vi "Get Lines Parameters.vi"(6 "P2 Y (unreleased)":refnum<class "1D Array f32.lvclass">, 8 "error in (no error)":errorcluster, 9 "P1 Y (unreleased)":refnum<class "1D Array f32.lvclass">, 10 "P2 X (unreleased)":refnum<class "1D Array f32.lvclass">, 11 "P1 X (unreleased)":refnum<class "1D Array f32.lvclass">) -> (0 "error out":errorcluster, 1 "Quadrant Correction X":refnum<class "1D Array f32.lvclass">, 2 "Direction Coefficients":refnum<class "1D Array f32.lvclass">, 3 "Quadrant Correction Y":refnum<class "1D Array f32.lvclass">, 5 "Length of Lines":refnum<class "1D Array f32.lvclass">, 7 "Is Row Major Line":refnum<class "1D Array binary.lvclass">)   [LabVIEW 2024, in "G2CPU Line Profile.lvlib"]
uses:
  G2CPU Line Profile.lvlib
  <vilib>/Natan Biesmans/G2CPU GPU and CPU HPC Toolkit/G2CPU Libraries/Arrays/1DArray/f32/1D Array f32.lvclass
  C:/Program Files/National Instruments/LabVIEW 2025/vi.lib/Natan Biesmans/G2CPU GPU and CPU HPC Toolkit/G2CPU Libraries/Arrays/Array/Array Prototype.lvclass
  <vilib>/Natan Biesmans/G2CPU GPU and CPU HPC Toolkit/G2CPU Libraries/Arrays/1DArray/binary/1D Array binary.lvclass
  cbe0f89a-fc6c-489f-bd70-ceba54479500.vi
  1a5ec087-74ba-4451-afc4-8685a5b5da5b.vi
  39281530-9ad4-4b96-9f34-9893a8ab4de5.vi
  7e7af70b-50f8-473b-bd23-2dd50eabd212.vi
  0e1627f4-ff60-46ab-8acd-18b1de2a0878.vi
  0517fff0-634e-4db0-931a-045051f9f055.vi
  a74614b9-8be0-4acb-b2b7-f56f2ea25a1a.vi
  cbe0f89a-fc6c-489f-bd70-ceba54479500.vi/1bf6e03b-eb75-45f6-9764-49dc38a3a024.vi
  cbe0f89a-fc6c-489f-bd70-ceba54479500.vi/2da4419f-02df-47a7-be00-1b7e0871fa33.vi
  1a5ec087-74ba-4451-afc4-8685a5b5da5b.vi/1bf6e03b-eb75-45f6-9764-49dc38a3a024.vi
  1a5ec087-74ba-4451-afc4-8685a5b5da5b.vi/2da4419f-02df-47a7-be00-1b7e0871fa33.vi
  39281530-9ad4-4b96-9f34-9893a8ab4de5.vi/def40612-844c-421c-bb75-87c330777b0b.vi
  7e7af70b-50f8-473b-bd23-2dd50eabd212.vi/def40612-844c-421c-bb75-87c330777b0b.vi
  0e1627f4-ff60-46ab-8acd-18b1de2a0878.vi/46771f49-eb1d-473b-8e81-f516cef50a4e.vi
  0e1627f4-ff60-46ab-8acd-18b1de2a0878.vi/dc76f8e4-64fa-456a-8549-7a4b6936c4c9.vi
  0e1627f4-ff60-46ab-8acd-18b1de2a0878.vi/7e60ddfb-e748-4c0c-85da-e395a1b7978d.vi
  0e1627f4-ff60-46ab-8acd-18b1de2a0878.vi/d2eceff7-f641-4ce4-acfa-e9e293a3c877.vi
  0e1627f4-ff60-46ab-8acd-18b1de2a0878.vi/b737122b-4036-448b-abd3-e2701355e828.vi
  0517fff0-634e-4db0-931a-045051f9f055.vi/494f1156-cf2e-4254-b6af-02aaeb6c0aff.vi
  0517fff0-634e-4db0-931a-045051f9f055.vi/44c17688-3442-4a50-bd81-3405ead58fa2.vi
  a74614b9-8be0-4acb-b2b7-f56f2ea25a1a.vi/b114fc2c-bc52-4e9d-afcd-b3046867ff8e.vi
  a74614b9-8be0-4acb-b2b7-f56f2ea25a1a.vi/ad131c31-fa70-445f-95fa-04e91a18ad4e.vi
  cbe0f89a-fc6c-489f-bd70-ceba54479500.vi/1bf6e03b-eb75-45f6-9764-49dc38a3a024.vi/3e802c67-fb96-46a3-ae13-4994a8508b4f.vi
  cbe0f89a-fc6c-489f-bd70-ceba54479500.vi/1bf6e03b-eb75-45f6-9764-49dc38a3a024.vi/5a50fc67-79e7-4972-80c2-92243cd53dd4.vi
  cbe0f89a-fc6c-489f-bd70-ceba54479500.vi/2da4419f-02df-47a7-be00-1b7e0871fa33.vi/730f6c57-5c0b-4ee9-b61e-75067b25222b.vi
  cbe0f89a-fc6c-489f-bd70-ceba54479500.vi/2da4419f-02df-47a7-be00-1b7e0871fa33.vi/096b8799-7810-404e-baca-ba9279cec4bd.vi
  cbe0f89a-fc6c-489f-bd70-ceba54479500.vi/2da4419f-02df-47a7-be00-1b7e0871fa33.vi/0f1a5a47-bcc5-4796-ac31-8dfcfbc0d7d1.vi
  cbe0f89a-fc6c-489f-bd70-ceba54479500.vi/2da4419f-02df-47a7-be00-1b7e0871fa33.vi/89f12e17-3330-4b72-ad8f-8dd636660732.vi
  1a5ec087-74ba-4451-afc4-8685a5b5da5b.vi/1bf6e03b-eb75-45f6-9764-49dc38a3a024.vi/3e802c67-fb96-46a3-ae13-4994a8508b4f.vi
  1a5ec087-74ba-4451-afc4-8685a5b5da5b.vi/1bf6e03b-eb75-45f6-9764-49dc38a3a024.vi/5a50fc67-79e7-4972-80c2-92243cd53dd4.vi
  1a5ec087-74ba-4451-afc4-8685a5b5da5b.vi/2da4419f-02df-47a7-be00-1b7e0871fa33.vi/730f6c57-5c0b-4ee9-b61e-75067b25222b.vi
  1a5ec087-74ba-4451-afc4-8685a5b5da5b.vi/2da4419f-02df-47a7-be00-1b7e0871fa33.vi/096b8799-7810-404e-baca-ba9279cec4bd.vi
  1a5ec087-74ba-4451-afc4-8685a5b5da5b.vi/2da4419f-02df-47a7-be00-1b7e0871fa33.vi/0f1a5a47-bcc5-4796-ac31-8dfcfbc0d7d1.vi
  1a5ec087-74ba-4451-afc4-8685a5b5da5b.vi/2da4419f-02df-47a7-be00-1b7e0871fa33.vi/89f12e17-3330-4b72-ad8f-8dd636660732.vi
  0e1627f4-ff60-46ab-8acd-18b1de2a0878.vi/dc76f8e4-64fa-456a-8549-7a4b6936c4c9.vi/3e802c67-fb96-46a3-ae13-4994a8508b4f.vi
  0e1627f4-ff60-46ab-8acd-18b1de2a0878.vi/dc76f8e4-64fa-456a-8549-7a4b6936c4c9.vi/5a50fc67-79e7-4972-80c2-92243cd53dd4.vi
  0517fff0-634e-4db0-931a-045051f9f055.vi/494f1156-cf2e-4254-b6af-02aaeb6c0aff.vi/edd31282-7992-4bba-af75-482693dee5e1.vi
  a74614b9-8be0-4acb-b2b7-f56f2ea25a1a.vi/b114fc2c-bc52-4e9d-afcd-b3046867ff8e.vi/edd31282-7992-4bba-af75-482693dee5e1.vi
  a74614b9-8be0-4acb-b2b7-f56f2ea25a1a.vi/ad131c31-fa70-445f-95fa-04e91a18ad4e.vi/730f6c57-5c0b-4ee9-b61e-75067b25222b.vi
  a74614b9-8be0-4acb-b2b7-f56f2ea25a1a.vi/ad131c31-fa70-445f-95fa-04e91a18ad4e.vi/096b8799-7810-404e-baca-ba9279cec4bd.vi
  a74614b9-8be0-4acb-b2b7-f56f2ea25a1a.vi/ad131c31-fa70-445f-95fa-04e91a18ad4e.vi/0f1a5a47-bcc5-4796-ac31-8dfcfbc0d7d1.vi
  a74614b9-8be0-4acb-b2b7-f56f2ea25a1a.vi/ad131c31-fa70-445f-95fa-04e91a18ad4e.vi/89f12e17-3330-4b72-ad8f-8dd636660732.vi
  <vilib>/Natan Biesmans/G2CPU GPU and CPU HPC Toolkit/G2CPU Libraries/Arrays/SubVI/Lock Arrays.vi
  <vilib>/Natan Biesmans/G2CPU GPU and CPU HPC Toolkit/G2CPU Libraries/Arrays/Array/G2CPU Get Array Pointer.vi
  <vilib>/Natan Biesmans/G2CPU GPU and CPU HPC Toolkit/G2CPU Libraries/Arrays/SubVI/is 1D.vi
  <vilib>/Natan Biesmans/G2CPU GPU and CPU HPC Toolkit/ArrayFire Driver/VIs/sub.vi
  <vilib>/Natan Biesmans/G2CPU GPU and CPU HPC Toolkit/G2CPU Libraries/Arrays/Array/G2CPU Set Array Pointer.vi
  <vilib>/Natan Biesmans/G2CPU GPU and CPU HPC Toolkit/G2CPU Libraries/Arrays/Array/G2CPU Unlock Array.vi
  <vilib>/Natan Biesmans/G2CPU GPU and CPU HPC Toolkit/G2CPU Libraries/Arrays/Array/G2CPU Release Array.vi
  <vilib>/Natan Biesmans/G2CPU GPU and CPU HPC Toolkit/G2CPU Libraries/Arrays/Array/G2CPU Lock Array.vi
  <vilib>/Natan Biesmans/G2CPU GPU and CPU HPC Toolkit/ArrayFire Driver/VIs/abs.vi
  <vilib>/Natan Biesmans/G2CPU GPU and CPU HPC Toolkit/ArrayFire Driver/VIs/div.vi
  <vilib>/Natan Biesmans/G2CPU GPU and CPU HPC Toolkit/ArrayFire Driver/VIs/gt.vi
  <vilib>/Natan Biesmans/G2CPU GPU and CPU HPC Toolkit/ArrayFire Driver/VIs/maxof.vi
  <vilib>/Natan Biesmans/G2CPU GPU and CPU HPC Toolkit/G2CPU Libraries/Arrays/Array/Array Prototype.lvclass
  <vilib>/Natan Biesmans/G2CPU GPU and CPU HPC Toolkit/G2CPU Libraries/Arrays/DataTypes/f32/f32.lvclass
  <vilib>/Natan Biesmans/G2CPU GPU and CPU HPC Toolkit/G2CPU Libraries/Arrays/1DArray/1D Array Prototype.lvclass
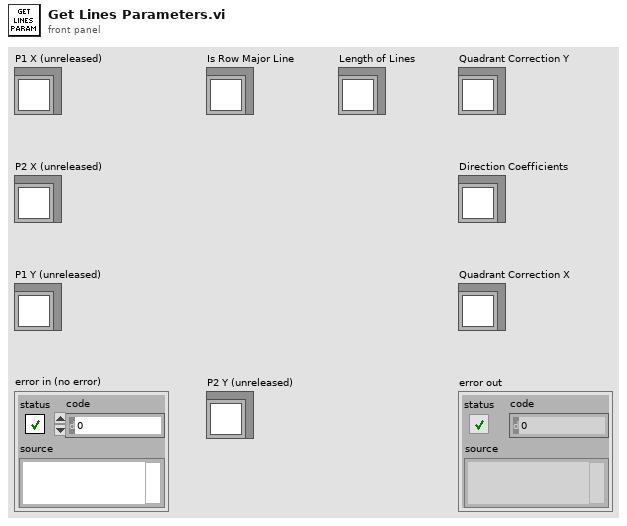
[diagram p1: front panel]
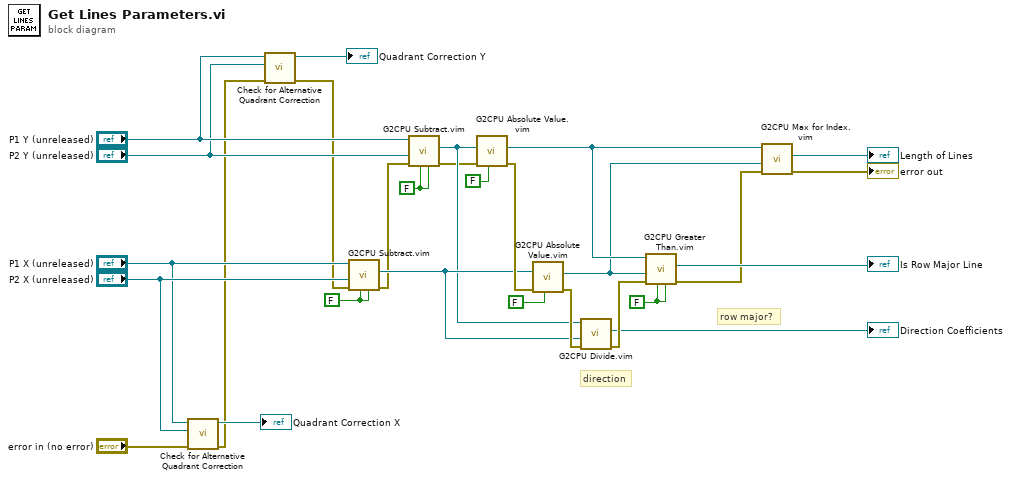
[diagram p0: block diagram]
diagram:
  w1 = FALSE ("Auto Release lhs (Enabled)")
  w2 = FALSE ("Auto Release lhs (Enabled)")
  w18 = FALSE ("Auto Release lhs (Enabled)")
  # "row major?"
  # "direction"
  n1 = call "Check for Alternative Quadrant Correction.vi"("error in (no error)"="error in (no error)", "End Point (unreleased)"="P2 X (unreleased)", "Starting Point (unreleased)"="P1 X (unreleased)") -> ("error out"=w4:errorcluster, "Quadrant Correction"=→"Quadrant Correction X":refnum<class "1D Array f32.lvclass">)  [unwired: 7 in]
  n2 = call "Check for Alternative Quadrant Correction.vi"("error in (no error)"=w4, "End Point (unreleased)"="P2 Y (unreleased)", "Starting Point (unreleased)"="P1 Y (unreleased)") -> ("error out"=w5:errorcluster, "Quadrant Correction"=→"Quadrant Correction Y":refnum<class "1D Array f32.lvclass">)  [unwired: 7 in]
  n3 = call "G2CPU Subtract.vim"("Auto Release rhs (Enabled)"=w2, "Auto Release lhs (Enabled)"=w2, "error in (no error)"=w5, "Array rhs"="P2 X (unreleased)", "Array lhs"="P1 X (unreleased)") -> ("error out"=w6:errorcluster, "Array Result"=w9:refnum<class "1D Array f32.lvclass">)  [unwired: 5 in]
  n4 = call "G2CPU Subtract.vim"("Auto Release rhs (Enabled)"=w1, "Auto Release lhs (Enabled)"=w1, "error in (no error)"=w6, "Array rhs"="P2 Y (unreleased)", "Array lhs"="P1 Y (unreleased)") -> ("error out"=w7:errorcluster, "Array Result"=w8:refnum<class "1D Array f32.lvclass">)  [unwired: 5 in]
  n5 = call "G2CPU Absolute Value.vim"("Auto Release (Enabled)"=FALSE, "error in (no error)"=w7, "Array in"=w8) -> ("error out"=w11:errorcluster, "Array Result"=w15:refnum<class "1D Array f32.lvclass">)  [unwired: 7 in]
  n6 = call "G2CPU Absolute Value.vim"("Auto Release (Enabled)"=FALSE, "error in (no error)"=w11, "Array in"=w9) -> ("error out"=w10:errorcluster, "Array Result"=w14:refnum<class "1D Array f32.lvclass">)  [unwired: 7 in]
  n7 = call "G2CPU Divide.vim"("error in (no error)"=w10, "Array rhs"=w9, "Array lhs"=w8) -> ("error out"=w21:errorcluster, "Array Result"=→"Direction Coefficients":refnum<class "1D Array f32.lvclass">)  [unwired: 7 in]
  n8 = call "G2CPU Greater Than.vim"("Auto Release rhs (Enabled)"=w18, "Auto Release lhs (Enabled)"=w18, "error in (no error)"=w21, "Array rhs"=w14, "Array lhs"=w15) -> ("error out"=w16:errorcluster, "Array Result"=→"Is Row Major Line":refnum<class "1D Array binary.lvclass">)  [unwired: 5 in]
  n9 = call "G2CPU Max for Index.vim"("error in (no error)"=w16, "Array rhs"=w14, "Array lhs"=w15) -> ("error out"=→"error out":errorcluster, "Array Result"=→"Length of Lines":refnum<class "1D Array f32.lvclass">)  [unwired: 7 in]
